vi "d_encoder_test_ramp.vi"() -> ()   [LabVIEW 2014]
uses:
  <vilib>/eio/EIONode/EIONode.xnode
  <vilib>/rvi/FXPMathLib/FxpMul/XNode/nifxpmath_Multiplier.xnode
  <vilib>/rvi/FXPMathLib/sim/FxpSim.dll
  <vilib>/rvi/eio/common/nirviEmuTemplateMethod_errors.vi
  <vilib>/rvi/FXPMathLib/FxpSinAndCos/XNode/nifxpmath_SinAndCos.xnode
  <vilib>/rvi/FXPMathLib/FxpSinAndCos/simVIs/DllFxpSinAndCosTemp_sub.vi
  <vilib>/rvi/FXPMathLib/FxpSinAndCos/subVIs/nifxpmath_SinAndCos_SimConfig.ctl
  <vilib>/rvi/Analysis/measure/butterworth/XNode/niFpgaButterworthFilter.xnode
  <vilib>/rvi/FXPMathLib/FxpSub/XNode/nifxpmath_Sub.xnode
  <vilib>/rvi/FXPMathLib/FxpAdd/XNode/nifxpmath_Add.xnode
  <vilib>/rvi/DataTransferAndStorage/Container/XNode/niFpgaContainer.xnode
  <vilib>/rvi/interface/RandomDataEmulation/nirviRandomDataFpgaMultiElementTemplate.vi
panel:
  out "Dr":fxp<+/-,64,20>
  in  "Step / Ramp":bool
  out "Dr_ramp":fxp<+/-,64,20>
  out "D_slope":fxp<+/-,32,6>
  in  "D_time":fxp<+/-,41,11>
  in  "D_end":fxp<+/-,22,7>
  in  "Ramp start":bool
  out "time now (s)":fxp<+,52,14>
  out "D_i":fxp<+/-,34,18>
  in  "D_tolorence":fxp<+/-,14,3>
  in  "Ki":fxp<+/-,20,6>
  out "D_error":fxp<+/-,24,11>
  in  "Direction":bool
  out "Fmr_PD":fxp<+/-,64,31>
  in  "Kd":fxp<+/-,20,8>
  in  "Kp":fxp<+/-,20,12>
  in  "scaled coefficients_D_dd":i32[](array[numeric])=[780119100, 146811362]
  out "D_dd":fxp<+/-,36,29>
  in  "Ini coe.":bool
  out "va":fxp<+/-,38,8>
  out "vb":fxp<+/-,38,8>
  in  "stop motor":bool
  out "vq_F":fxp<+/-,20,5> format="%.57g"
  out "vd_F":fxp<+/-,20,5>
  out "D_d (mm/s)":fxp<+/-,32,12>
  out "mt":u32
  out "omega (rad/s)":fxp<+/-,32,18>
  in  "mt0":u32
  out "D(mm)":fxp<+/-,22,7>
  out "rad(NrTheta)":fxp<+/-,33,18>
  out "Encoder Position":i32
  in  "Encoder Reset":bool
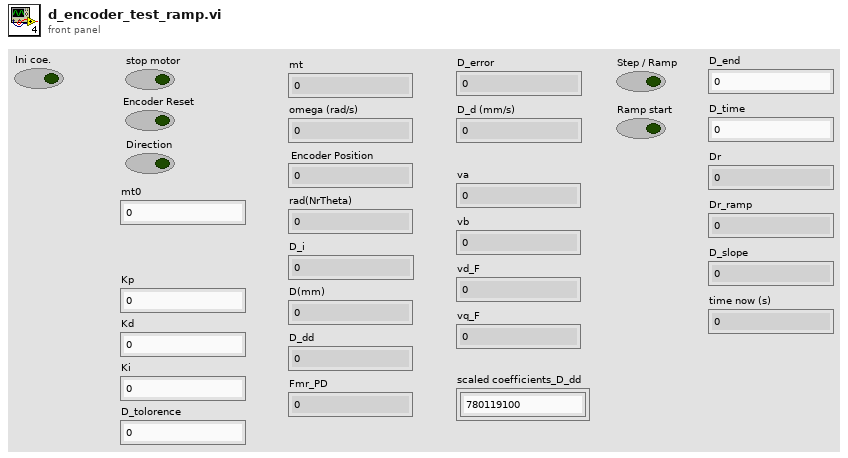
[diagram p1: front panel]
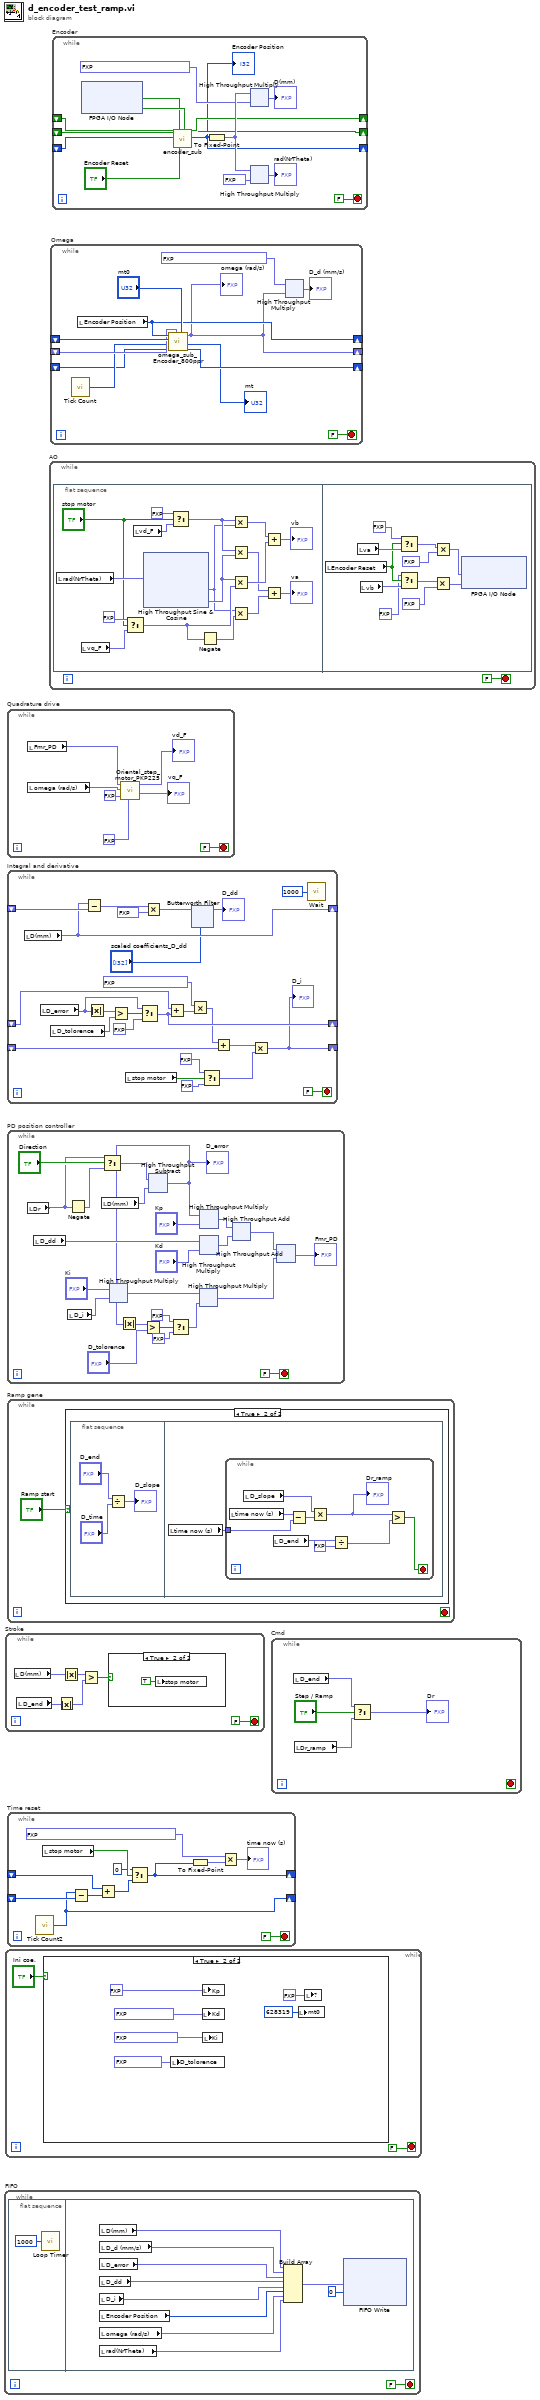
[diagram p0: block diagram]
diagram:
  n1 = while "FIFO" {
    stop <- FALSE stop-if-true
    n2 = flat-sequence {
      frame #0 {
        n3 = call "Loop Timer"("Count(uSec)"=u32 1000) -> ()  [unwired: 1 out]
      }
      frame #1 {
        n4 = local read "D(mm)"() -> (w10:fxp<+/-,22,7>)
        n5 = local read "D_d (mm/s)"() -> (w9:fxp<+/-,32,12>)
        n6 = local read "D_error"() -> (w8:fxp<+/-,24,11>)
        n7 = local read "D_dd"() -> (w7:fxp<+/-,36,29>)
        n8 = local read "D_i"() -> (w6:fxp<+/-,34,18>)
        n9 = local read "Encoder Position"() -> (w5:i32)
        n10 = local read "omega (rad/s)"() -> (w4:fxp<+/-,32,18>)
        n11 = local read "rad(NrTheta)"() -> (w3:fxp<+/-,33,18>)
        n12 = Build Array(w10, w9, w8, w7, w6, w5, w4, w3) -> (w11:fxp<+/-,52,32>[])
        n13 = xnode ("FIFO Write")("Element"=w11, "Timeout"=0) -> ()  [unwired: 1 in, 2 out]
      }
    }
  }
  n14 = while "Stroke" {
    stop <- FALSE stop-if-true
    n15 = local read "D(mm)"() -> (w18:fxp<+/-,22,7>)
    n16 = local read "D_end"() -> (w14:fxp<+/-,22,7>)
    n17 = Absolute Value(x=w14) -> (abs(x)=w13:fxp<+,22,7>)
    n18 = Absolute Value(x=w18) -> (abs(x)=w17:fxp<+,22,7>)
    n19 = Greater?(x=w17, y=w13) -> (0:w16:bool)
    n20 = case shown="True" w16 {
      frame False {
      }
      frame True {
        n21 = local write "stop motor"(TRUE ("stop motor")) -> ()
      }
    }
  }
  n22 = while {
    stop <- FALSE stop-if-true
    n23 = case shown="True" "Ini coe." {
      frame False {
      }
      frame True {
        n24 = local write "D_tolorence"(fxp<+/-,14,3> 0.009765625 ("D_tolorence")) -> ()
        n25 = local write "Kp"(fxp<+/-,20,12> 2.0 ("Kp")) -> ()
        n26 = local write "Kd"(fxp<+/-,20,8> 1.800048828125 ("Kd")) -> ()
        n27 = local write "Ki"(fxp<+/-,20,6> 0.0999755859375 ("D_i")) -> ()
        n28 = local write "mt0"(u32 628319 ("mt0")) -> ()
        n29 = local write item#-1(fxp<+/-,11,7> 20.0 ("Fmr")) -> ()
      }
    }
  }
  n30 = while "Quadrature drive" {
    stop <- FALSE stop-if-true
    n31 = local read "Fmr_PD"() -> (w28:fxp<+/-,64,31>)
    n32 = local read "omega (rad/s)"() -> (w30:fxp<+/-,32,18>)
    n33 = call "Oriental_step_motor_PKP225.vi"("F_Threshold"=fxp<+,12,12> 10.0, "dFmr"=fxp<+/-,25,15> 0.0, "omega"=w30, "Fmr"=w28) -> ("vq_F"=→"vq_F":fxp<+/-,20,5>, "vd_F"=→"vd_F":fxp<+/-,20,5>)  [unwired: 6 in]
  }
  n34 = while "Integral and derivative" {
    shift-right: [w55] -> _
    shift-left: _ -> [w59]
    shift-right: [w45] -> _
    shift-left: _ -> [w46]
    shift-right: [w35] -> _
    shift-left: _ -> [w39]
    stop <- FALSE stop-if-true
    n35 = local read "D(mm)"() -> (w55:fxp<+/-,22,7>)
    n36 = local read "D_error"() -> (w47:fxp<+/-,24,11>)
    n37 = local read "D_tolorence"() -> (w50:fxp<+/-,14,3>)
    n38 = Subtract(x=w55, y=w59) -> (x-y=w58:fxp<+/-,23,8>)
    n39 = Absolute Value(x=w47) -> (abs(x)=w51:fxp<+,24,11>)
    n40 = Greater?(x=w51, y=w50) -> (0:w49:bool)
    n41 = local read "stop motor"() -> (w42:bool)
    n42 = Select(t=w47, s=w49, f=fxp<+,24,11> 0.0) -> (s? t:f=w45:fxp<+/-,25,12>)
    n43 = Multiply(x=w58, y=fxp<+/-,33,13> 1000.0) -> (x*y=w56:fxp<+/-,55,20>)
    n44 = Add(x=w46, y=w45) -> (x+y=w44:fxp<+/-,26,13>)
    n45 = Multiply(x=fxp<+/-,30,12> 0.000499725341796875, y=w44) -> (x*y=w38:fxp<+/-,55,24>)
    n46 = xnode "Butterworth Filter"("input data"=w56, "scaled coefficients"="scaled coefficients_D_dd") -> ("output data"=→"D_dd":fxp<+/-,36,24>)  [unwired: 1 in]
    n47 = Select(t=fxp<+,1,1> 0.0, s=w42, f=fxp<+,1,1> 1.0) -> (s? t:f=w36:fxp<+,1,1>)
    n48 = Add(x=w38, y=w39) -> (x+y=w37:fxp<+/-,32,16>)
    n49 = Multiply(x=w37, y=w36) -> (x*y=w35:fxp<+/-,32,16>)
    "D_i" <- w35
    n50 = call "Wait"("Count(uSec)"=u32 1000) -> ()  [unwired: 1 out]
  }
  n51 = while "PD position controller" {
    stop <- FALSE stop-if-true
    n52 = local read "Dr"() -> (w69:fxp<+/-,64,20>)
    n53 = local read "D_dd"() -> (w88:fxp<+/-,36,29>)
    n54 = local read "D_i"() -> (w80:fxp<+/-,34,18>)
    n55 = Negate(x=w69) -> (-x=w84:fxp<+/-,64,21>)
    n56 = local read "D(mm)"() -> (w92:fxp<+/-,22,7>)
    n57 = Select(t=w69, s="Direction", f=w84) -> (s? t:f=w83:fxp<+/-,64,21>)
    n58 = xnode ("High Throughput Multiply")("x"="Ki", "y"=w80) -> ("x*y"=w74:fxp<+/-,54,24>)
    n59 = xnode "High Throughput Subtract"("x"=w83, "y"=w92) -> ("x-y"=w78:fxp<+/-,64,22>)
    "D_error" <- w78
    n60 = Absolute Value(x=w78) -> (abs(x)=w79:fxp<+,64,22>)
    n61 = Greater?(x=w79, y="D_tolorence") -> (0:w77:bool)
    n62 = Select(t=fxp<+,10,2> 1.0, s=w77, f=fxp<+,10,2> 0.0) -> (s? t:f=w73:fxp<+,10,2>)
    n63 = xnode ("High Throughput Multiply")("x"=w74, "y"=w73) -> ("x*y"=w70:fxp<+/-,64,26>)
    n64 = xnode ("High Throughput Multiply")("x"=w78, "y"="Kp") -> ("x*y"=w90:fxp<+/-,64,34>)
    n65 = xnode ("High Throughput Multiply")("x"=w88, "y"="Kd") -> ("x*y"=w89:fxp<+/-,56,37>)
    n66 = xnode ("High Throughput Add")("x"=w90, "y"=w89) -> ("x+y"=w71:fxp<+/-,64,38>)
    n67 = xnode ("High Throughput Add")("x"=w71, "y"=w70) -> ("x+y"=→"Fmr_PD":fxp<+/-,64,39>)
  }
  n68 = while "Ramp gene" {
    stop <- _ stop-if-true
    n69 = case shown="True" "Ramp start" {
      frame False {
      }
      frame True {
        n70 = flat-sequence {
          frame #0 {
            n71 = Divide(x="D_end", y="D_time") -> (x/y=→"D_slope":fxp<+/-,64,38>)
          }
          frame #1 {
            n72 = local read "time now (s)"() -> (w97:fxp<+,52,14>)
            n73 = while {
              tunnel: w97 -> [w105]
              stop <- w101 stop-if-true
              n74 = local read "time now (s)"() -> (w106:fxp<+,52,14>)
              n75 = local read "D_slope"() -> (w103:fxp<+/-,32,6>)
              n76 = local read "D_end"() -> (w100:fxp<+/-,22,7>)
              n77 = Subtract(x=w106, y=w105) -> (x-y=w104:fxp<+/-,53,15>)
              n78 = Multiply(x=w103, y=w104) -> (x*y=w102:fxp<+/-,64,20>)
              "Dr_ramp" <- w102
              n79 = Divide(x=w100, y=fxp<+/-,22,7> 2.0) -> (x/y=w98:fxp<+/-,45,23>)
              n80 = Greater?(x=w102, y=w98) -> (0:w101:bool)
            }
          }
        }
      }
    }
  }
  n81 = while "Time reset" {
    shift-right: [w111] -> _
    shift-left: _ -> [w116]
    shift-right: [w112] -> _
    shift-left: _ -> [w117]
    stop <- FALSE stop-if-true
    n82 = call "Tick Count2"() -> ("Tick Count(uSec)"=w112:u32)
    n83 = local read "stop motor"() -> (w114:bool)
    n84 = Subtract(x=w112, y=w117) -> (x-y=w118:u32)
    n85 = Add(x=w116, y=w118) -> (x+y=w115:u32)
    n86 = Select(t=u32 0, s=w114, f=w115) -> (s? t:f=w111:u32)
    n87 = To Fixed-Point(number=w111) -> (fixed-point=w110:fxp<+,32,32>)  [unwired: 1 in]
    n88 = Multiply(x=fxp<+,20,-18> 1.0000003385357559e-06, y=w110) -> (x*y=→"time now (s)":fxp<+,52,14>)
  }
  n89 = while "AO" {
    stop <- FALSE stop-if-true
    n90 = flat-sequence {
      frame #0 {
        n91 = local read "rad(NrTheta)"() -> (w135:fxp<+/-,33,18>)
        n92 = local read "vq_F"() -> (w133:fxp<+/-,20,5>)
        n93 = Select(t=fxp<+,20,5> 0.0, s="stop motor", f=w133) -> (s? t:f=w130:fxp<+/-,21,6>)
        n94 = local read "vd_F"() -> (w134:fxp<+/-,20,5>)
        n95 = xnode "High Throughput Sine & Cosine"("x (pi)"=w135) -> ("sin(x)"=w126:fxp<+/-,17,2>, "cos(x)"=w128:fxp<+/-,17,2>)
        n96 = Select(t=fxp<+,20,5> 0.0, s="stop motor", f=w134) -> (s? t:f=w127:fxp<+/-,21,6>)
        n97 = Negate(x=w130) -> (-x=w129:fxp<+/-,21,6>)
        n98 = Multiply(x=w127, y=w126) -> (x*y=w125:fxp<+/-,37,7>)
        n99 = Multiply(x=w127, y=w128) -> (x*y=w123:fxp<+/-,37,7>)
        n100 = Multiply(x=w128, y=w130) -> (x*y=w124:fxp<+/-,37,7>)
        n101 = Multiply(x=w126, y=w129) -> (x*y=w122:fxp<+/-,37,7>)
        n102 = Add(x=w125, y=w124) -> (x+y=→"vb":fxp<+/-,38,8>)
        n103 = Add(x=w123, y=w122) -> (x+y=→"va":fxp<+/-,38,8>)
      }
      frame #1 {
        n104 = local read "Encoder Reset"() -> (w169:bool)
        n105 = local read "va"() -> (w171:fxp<+/-,38,8>)
        n106 = local read "vb"() -> (w170:fxp<+/-,38,8>)
        n107 = Select(t=fxp<+/-,20,5> 5.0 ("y"), s=w169, f=w171) -> (s? t:f=w172:fxp<+/-,38,8>)
        n108 = Select(t=fxp<+/-,20,5> 0.0 ("y"), s=w169, f=w170) -> (s? t:f=w173:fxp<+/-,38,8>)
        n109 = Multiply(x=w173, y=fxp<+/-,20,5> -0.5) -> (x*y=w177:fxp<+/-,57,12>)
        n110 = Multiply(x=w172, y=fxp<+/-,20,5> -0.5) -> (x*y=w176:fxp<+/-,57,12>)
        n111 = xnode "FPGA I/O Node"("Mod8/AO0"=w176, "Mod8/AO1"=w177) -> ()  [unwired: 2 in, 2 out]
      }
    }
  }
  n112 = while "Omega" {
    shift-right: [w187] -> _
    shift-left: _ -> [w188]
    shift-right: [w180] -> _
    shift-left: _ -> [w186]
    shift-right: [w183] -> _
    shift-left: _ -> [w184]
    stop <- FALSE stop-if-true
    n113 = call "Tick Count"() -> ("Tick Count(Ticks)"=w185:u32)
    n114 = local read "Encoder Position"() -> (w187:i32)
    n115 = call "omega_sub_Encoder_800ppr.vi"("mt0"="mt0", "omega_pre"=w186, "ticks_m_pre"=w184, "ticks"=w185, "count_pre"=w188, "count"=w187) -> ("ticks_m"=w183:u32, "mt"=→"mt":u32, "omega"=w180:fxp<+/-,20,9>)  [unwired: 3 in]
    "omega (rad/s)" <- w180
    n116 = xnode ("High Throughput Multiply")("x"=fxp<+/-,26,1> 0.3183099031448364, "y"=w180) -> ("x*y"=→"D_d (mm/s)":fxp<+/-,46,10>)
  }
  n117 = while "Encoder" {
    shift-right: [w196] -> _
    shift-left: _ -> [w198]
    shift-right: [w195] -> _
    shift-left: _ -> [w197]
    shift-right: [w193] -> _
    shift-left: _ -> [w194]
    stop <- FALSE stop-if-true
    n118 = xnode "FPGA I/O Node"() -> ("Mod4/DI3"=w203:bool, "Mod4/DI4"=w204:bool)  [unwired: 2 in, 2 out]
    n119 = call "encoder_sub.vi"("A_pre"=w198, "B_pre"=w197, "Encoder Position_pre"=w194, "A input"=w203, "Encoder Position Reset"="Encoder Reset", "B input"=w204) -> ("A"=w196:bool, "B"=w195:bool, "Encoder Position (Counts)"=w193:i32)  [unwired: 19 in]
    "Encoder Position" <- w193
    n120 = To Fixed-Point(number=w193) -> (fixed-point=w201:fxp<+/-,32,32>)  [unwired: 1 in]
    n121 = xnode ("High Throughput Multiply")("x"=w201, "y"=fxp<+/-,24,0> 0.002499997615814209) -> ("x*y"=→"D(mm)":fxp<+/-,56,32>)
    n122 = xnode ("High Throughput Multiply")("x"=w201, "y"=fxp<+/-,24,0> 0.125) -> ("x*y"=→"rad(NrTheta)":fxp<+/-,56,32>)
  }
  n123 = while "Cmd" {
    stop <- _ stop-if-true
    n124 = local read "D_end"() -> (w206:fxp<+/-,22,7>)
    n125 = local read "Dr_ramp"() -> (w205:fxp<+/-,64,20>)
    n126 = Select(t=w206, s="Step / Ramp", f=w205) -> (s? t:f=→"Dr":fxp<+/-,64,20>)
  }
